vi "SSH_TUNNEL_RemotePortToLocalPortConverter.vi"(8 "error in (no error)":errorcluster, 10 "Remote Port Number":u16, 11 "SSH_TUNNEL in":refnum<class "SSH_TUNNEL.lvclass">) -> (0 "error out":errorcluster, 2 "Local Port Number":u16, 3 "SSH_TUNNEL out":refnum<class "SSH_TUNNEL.lvclass">)   [LabVIEW 2018, in "SSH_TUNNEL.lvclass"]
uses:
  SSH_TUNNEL.lvclass
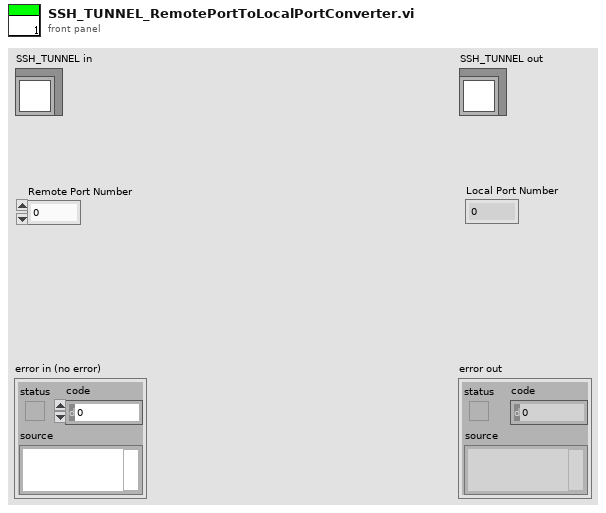
[diagram p1: front panel]
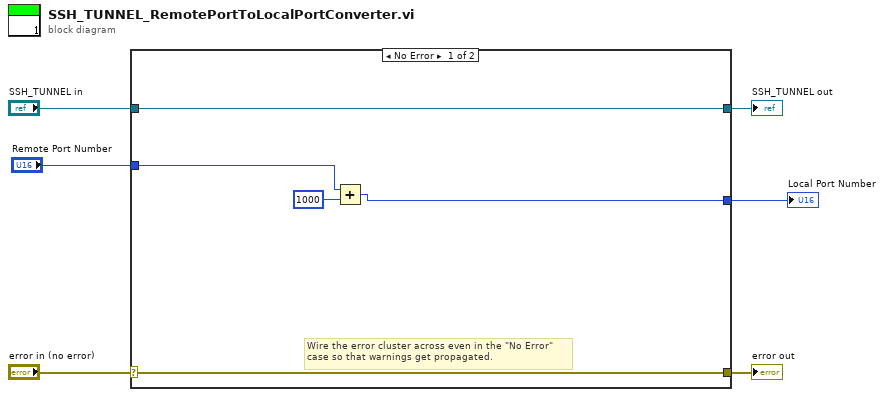
[diagram p0: block diagram]
diagram:
  n1 = case shown="No Error" "error in (no error)" {
    selector: "error in (no error)" -> [w10 w13]
    tunnel: [w10 w13] -> w5
    tunnel: [w11 w12] -> w3
    tunnel: "SSH_TUNNEL in" -> [w11 w12]
    tunnel: "Remote Port Number" -> [w9 _]
    tunnel: [w7 _] -> w1
    frame No Error {
      # "Wire the error cluster across even in the \"No Error\"\ncase so that warnings get propagated."
      n2 = Add(x=w9, y=u16 1000) -> (x+y=w7:u16)
    }
    frame Error {
    }
  }
  "error out" <- w5
  "SSH_TUNNEL out" <- w3
  "Local Port Number" <- w1
